vi "BLVac_readback.vi"(11 "Readback array":string[](array[string])) -> (1 "4500 TC1 2":dbl, 2 "Beamline":string, 3 "4500 IG":dbl, 4 "Beamline TC1 (Torr) 2":string, 5 "4500 TC2":dbl, 6 "Beamline TC1 (Torr)":string)   [LabVIEW 2014]
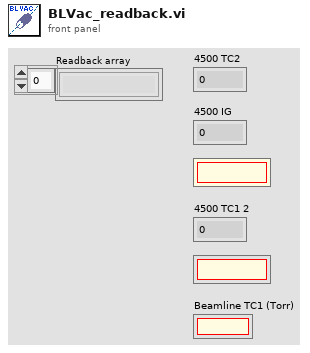
[diagram p1: front panel]
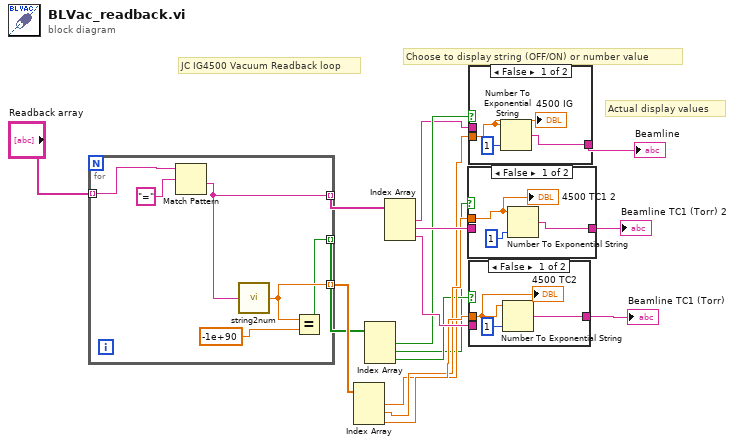
[diagram p0: block diagram]
diagram:
  # "JC IG4500 Vacuum Readback loop"
  # "Actual display values"
  # "Choose to display string (OFF/ON) or number value"
  n1 = for {
    tunnel: "Readback array" -> [w21] mode=indexing
    tunnel: [w17] -> w13 mode=indexing
    tunnel: [w19] -> w14 mode=indexing
    tunnel: [w20] -> w15 mode=indexing
    n2 = Match Pattern(string=w21, regular expression="=") -> (after substring=w17:string)  [unwired: 1 in, 3 out]
    n3 = call "string2num.vi"("string 2"=w17) -> ("Result"=w20:dbl)  [unwired: 8 in]
    n4 = Equal?(x=w20, y=-1e+90) -> (x = y?=w19:bool)
  }
  n5 = Index Array(array=w15) -> (element #1=w6:dbl, element #2=w7:dbl, element #3=w8:dbl)  [unwired: 3 in]
  n6 = Index Array(array=w14) -> (element #1=w3:bool, element #2=w4:bool, element #3=w5:bool)  [unwired: 3 in]
  n7 = Index Array(array=w13) -> (element #1=w2:string, element #2=w9:string, element #3=w10:string)  [unwired: 3 in]
  n8 = case shown="False" w4 {
    tunnel: w7 -> [w23 _]
    tunnel: w9 -> [_ w26]
    tunnel: [w25 w26] -> w16
    frame False {
      n9 = Number To Exponential String(number=w23, precision (6)=i16 1) -> (E-format string=w25:string)  [unwired: 2 in]
      "4500 TC1 2" <- w23
    }
    frame True {
    }
  }
  "Beamline TC1 (Torr) 2" <- w16
  n10 = case shown="False" w3 {
    tunnel: w2 -> [_ w30]
    tunnel: w6 -> [w27 _]
    tunnel: [w29 w30] -> w12
    frame False {
      n11 = Number To Exponential String(number=w27, precision (6)=i16 1) -> (E-format string=w29:string)  [unwired: 2 in]
      "4500 IG" <- w27
    }
    frame True {
    }
  }
  "Beamline" <- w12
  n12 = case shown="False" w5 {
    tunnel: w8 -> [w31 _]
    tunnel: w10 -> [_ w34]
    tunnel: [w33 w34] -> w11
    frame False {
      n13 = Number To Exponential String(number=w31, precision (6)=i16 1) -> (E-format string=w33:string)  [unwired: 2 in]
      "4500 TC2" <- w31
    }
    frame True {
    }
  }
  "Beamline TC1 (Torr)" <- w11
